vi "Number of Tests Sockets.vi"() -> ()   [LabVIEW 2019, in "UnitTestEngine.lvlib"]
uses:
  UnitTestEngine.lvlib
panel:
  in  "Number of Tests Sockets":u8=1 min=1 max=4
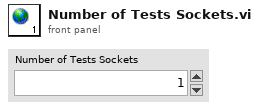
[diagram p1: front panel]
diagram:
